vi "Create Multiple 3D Plots 2012 NIVerified.vi"() -> ()   [LabVIEW 2019]
doc: "This VI uses a 3-D array of values to represent multiple plots and uses an ActiveX 3-D graph for displaying the plots."
uses:
  <vilib>/Platform/NI_3dgraph.lvlib
panel:
  in  "Plot Color Style":i32(ring)=1 items=["cwNone", "cwShaded", "cwColorSpectrum", "cwGrayScale", "cwCustom"]
  in  "Plot Colors":u32[](array[colorbox])=[16711680, 15706624, 16449346, 6618880, 16860]
  in  "3D Graph":refnum<k7>(container)
  # "Overview: This VI demonstrates how to graph multiple 3-D plots to the same graph indicator.\nRequirements: LabVIEW 2012 (or compatible)\nInstructions:\n1. Run the VI.\n2. Exercise the Plot Colors and Plot Color Style controls."
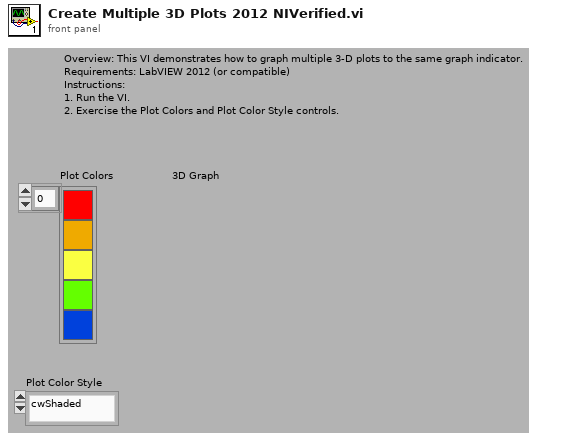
[diagram p1: front panel]
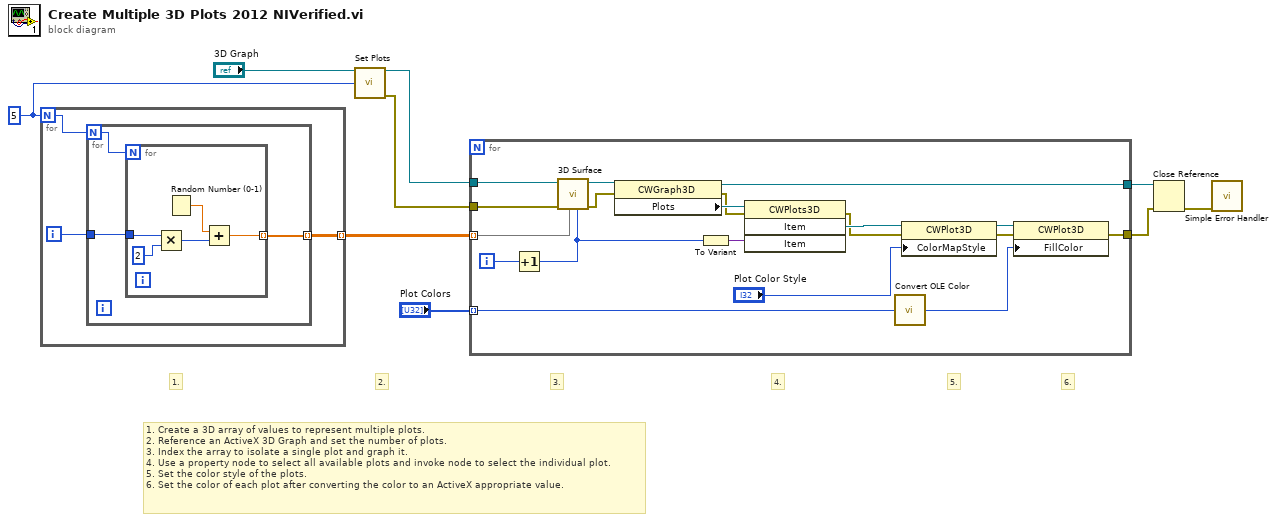
[diagram p0: block diagram]
diagram:
  w7 = 5
  # "1. Create a 3D array of values to represent multiple plots.\n2. Reference an ActiveX 3D Graph and set the number of plots.\n3. Index the array to isolate a single plot and graph it.\n4. Use a property node to select all available plots and invoke node to select the individual plot.\n5. Set the color style of the plots.\n6. Set the color of each plot after converting the color to an ActiveX appropriate value."
  # "6."
  # "5."
  # "4."
  # "3."
  # "2."
  # "1."
  n1 = for {
    N: w7 -> [w12]
    tunnel: [w10] -> w6 mode=indexing
    i -> [w11]
    n2 = for {
      N: w12 -> [w13]
      tunnel: w11 -> [w15]
      tunnel: [w14] -> w10 mode=indexing
      n3 = for {
        N: w13 -> [_]
        tunnel: w15 -> [w20]
        tunnel: [w16] -> w14 mode=indexing
        n4 = Multiply(x=w20, y=2) -> (x*y=w18:i32)
        n5 = Random Number (0-1)() -> (number: 0 to 1=w17:dbl)
        n6 = Add(x=w17, y=w18) -> (x+y=w16:dbl)
      }
    }
  }
  n7 = call <vilib>:"Set Plots.vi"("3D graph"="3D Graph", "# of plots(1)"=w7) -> ("3D graph out"=w5:refnum<k7>, "error out"=w8:errorcluster)  [unwired: 1 in, 11 out]
  n8 = for {
    tunnel: w8 -> [w39]
    tunnel: w5 -> [w38]
    tunnel: w6 -> [w36] mode=indexing
    tunnel: "Plot Colors" -> [w31] mode=indexing
    tunnel: [w23] -> w3
    tunnel: [w22] -> w2
    i -> [w37]
    n9 = Increment(x=w37) -> (x+1=w24:i32)
    n10 = call <vilib>:"3D Surface.vi"("plot number (1)"=w24, "z matrix"=w36, "error in (no error)"=w39, "3D graph"=w38) -> ("error out"=w34:errorcluster, "3D graph out"=w35:refnum<k7>)  [unwired: 6 out]
    n11 = property class="CWGraph3D"(reference=w35, error in=w34) -> (reference out=w23:refnum<k7>, error out=w32:errorcluster, "Plots"=w33:refnum<k7>)
    n12 = To Variant(anything=w24) -> (Variant=w25:variant)
    n13 = invoke class="CWPlots3D" method="Item"(reference=w33, error in=w32, "Item"=w25) -> (error out=w27:errorcluster, "Item"=w29:refnum<k7>)  [unwired: 1 in, 2 out]
    n14 = call <vilib>:"Convert OLE Color.vi"("color in"=w31) -> ("color out"=w30:u32)
    n15 = property class="CWPlot3D"(reference=w29, error in=w27, "ColorMapStyle"="Plot Color Style") -> (reference out=w28:refnum<k7>, error out=w26:errorcluster)
    n16 = property class="CWPlot3D"(reference=w28, error in=w26, "FillColor"=w30) -> (error out=w22:errorcluster)  [unwired: 1 out]
  }
  n17 = Close Reference(reference=w3, error in (no error)=w2) -> (error out=w1:errorcluster)
  n18 = call <vilib>:"Simple Error Handler.vi"("error in (no error)"=w1) -> ()  [unwired: 4 in, 5 out]
